vi "All Breaker Error Delay.vi"(9 "Delay (Ticks)":u32, 10 "Reset":bool, 11 "All Breakers Closed":bool) -> (2 "All Breaker Err Out":bool, 3 "Timer Running":bool)   [LabVIEW 2018]
doc: "Author: Scott Hannahs <sth@magnet.fsu.edu>\nCopyright 2018 Florida State University, All rights reserved."
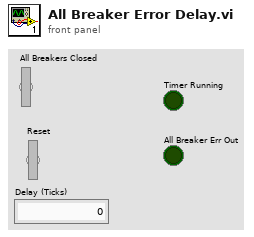
[diagram p1: front panel]
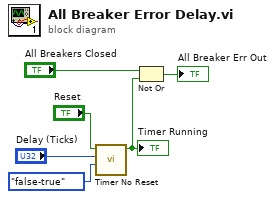
[diagram p0: block diagram]
diagram:
  n1 = call "Timer No Reset.vi"("Direction"=enum8{"either", "false-true", "true-false"}."false-true", "Tick Count(Ticks)"="Delay (Ticks)", "Start Timer"="Reset") -> ("Timer Running"=w1:bool)  [unwired: 8 in]
  "Timer Running" <- w1
  n2 = Not Or(1:w1, 2:"All Breakers Closed") -> (0:→"All Breaker Err Out":bool)
